vi "Get Node Class.vi"(8 "error in (no error)":errorcluster, 10 "Node Name":string, 11 "INI Deserializer in":refnum<class "INI Deserializer.lvclass">) -> (0 "error out":errorcluster, 2 "Node Class":string, 3 "INI Deserializer out":refnum<class "INI Deserializer.lvclass">)   [LabVIEW 2014, in "INI Deserializer.lvclass"]
uses:
  INI Deserializer.lvclass
  INI Deserializer.lvclass/INI Deserializer.ctl
  <vilib>/Utility/config.llb/Read Key (String).vi
  <vilib>/Utility/config.llb/NI_LVConfig.lvlib
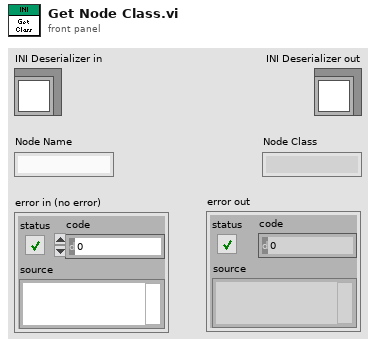
[diagram p1: front panel]
types:
  T1 = typedef "NI_LVConfig.lvlib/Config Data RefNum.ctl" = refnum<k1>
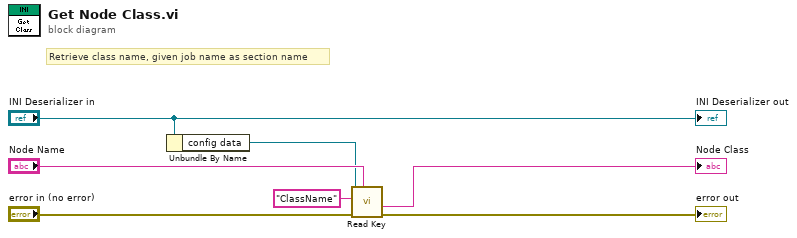
[diagram p0: block diagram]
diagram:
  # "Retrieve class name, given job name as section name"
  n1 = Unbundle By Name("INI Deserializer in") -> ("config data"=w1:T1)
  n2 = call-poly <vilib>:"Read Key.vi"("section"="Node Name", "error in (no error)"="error in (no error)", "key"="ClassName", "refnum"=w1) -> ("error out"=→"error out":errorcluster, "value"=→"Node Class":string)  [unwired: 4 in, 2 out]
  "INI Deserializer out" <- "INI Deserializer in"
